vi "processMsg.vi"(8 "error in (no error)":errorcluster, 10 "Refs":refnum<vi>[](array[refnum]), 11 "Msg in":string) -> (0 "error out":errorcluster, 3 "Msg out":string)   [LabVIEW 2017]
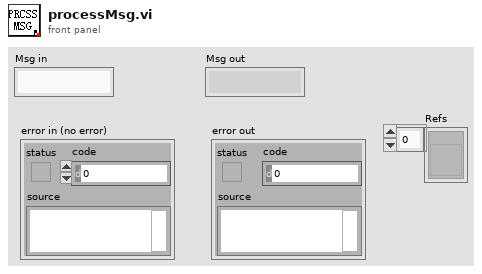
[diagram p1: front panel]
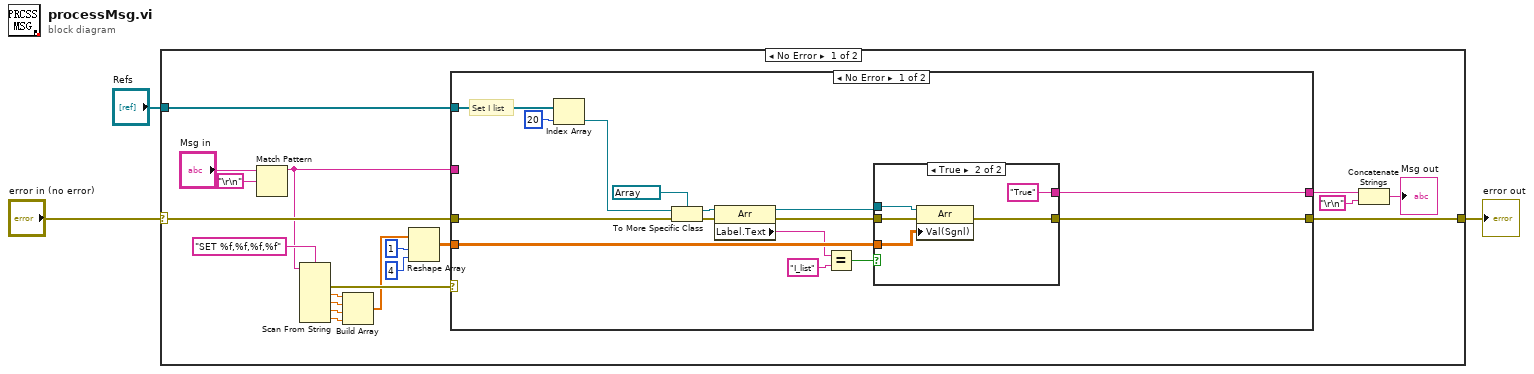
[diagram p0: block diagram]
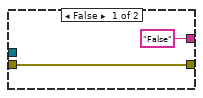
[diagram p2: hidden frame]
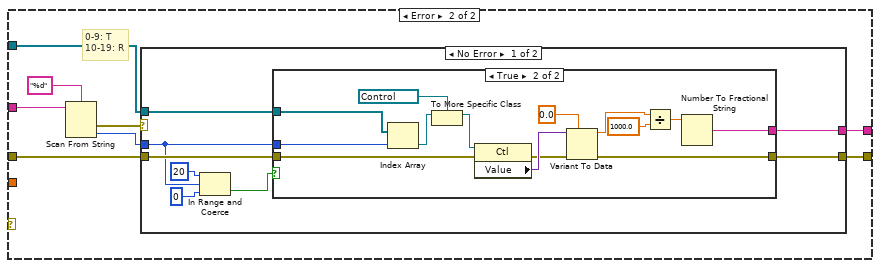
[diagram p3: hidden frame]
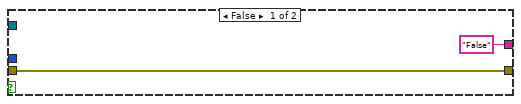
[diagram p4: hidden frame]
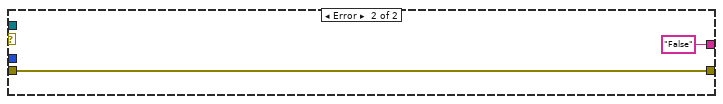
[diagram p5: hidden frame]
diagram:
  n1 = case shown="No Error" "error in (no error)" {
    selector: "error in (no error)" -> [w21 w79]
    tunnel: [w22 w79] -> w3
    tunnel: "Refs" -> [w15 _]
    frame No Error {
      n2 = Match Pattern(string="Msg in", regular expression="\r\n") -> (before substring=w17:string)  [unwired: 4 out]
      n3 = Scan From String(format string="SET %f,%f,%f,%f" ("regular expression"), input string=w17) -> (error out=w16:errorcluster, output 1=w14:dbl, output 2=w13:dbl, output 3=w12:dbl, output 4=w11:dbl)  [unwired: 6 in, 2 out]
      n4 = Build Array(w14, w13, w12, w11) -> (w10:dbl[])
      n5 = Reshape Array(w10, 1 ("dimension size"), 4 ("dimension size")) -> (w7:dbl[][])
      n6 = case shown="No Error" w16 {
        tunnel: [w23 w52] -> w22
        tunnel: w21 -> [w26 w47]
        tunnel: w17 -> [_ w49]
        tunnel: [w27 w51] -> w5
        tunnel: w15 -> [w37 w45]
        tunnel: w7 -> [w33 _]
        frame No Error {
          # "Set I list"
          n7 = Index Array(array=w37, index=20) -> (element=w34:refnum<vi>)
          n8 = To More Specific Class(target class=refnum<vi> refnum ("引用"), reference=w34, error in=w26) -> (specific class reference=w30:refnum<vi>, error out=w25:errorcluster)
          n9 = property class="Arr"(reference=w30, error in=w25) -> (reference out=w29:refnum<vi>, error out=w24:errorcluster, "Label.Text"=w31:string)
          n10 = Equal?(x=w31, y="I_list") -> (x = y?=w28:bool)
          n11 = case shown="True" w28 {
            tunnel: w33 -> [_ w44]
            tunnel: w29 -> [_ w43]
            tunnel: ["False" "True"] -> w27
            tunnel: w24 -> [w38 w41]
            tunnel: [w38 w40] -> w23
            frame False {
            }
            frame True {
              n12 = property class="Arr"(reference=w43, error in=w41, "Val(Sgnl)"=w44) -> (error out=w40:errorcluster)  [unwired: 1 out]
            }
          }
        }
        frame Error {
          # "0-9: T\n10-19: R"
          n13 = Scan From String(format string="%d" ("regular expression"), input string=w49) -> (error out=w48:errorcluster, output 1=w46:i32)  [unwired: 3 in, 2 out]
          n14 = case shown="No Error" w48 {
            tunnel: [w60 w78] -> w52
            tunnel: w47 -> [w59 w78]
            tunnel: [w58 "False" ("T (K) or R")] -> w51
            tunnel: w46 -> [w54 _]
            tunnel: w45 -> [w55 _]
            frame No Error {
              n15 = In Range and Coerce(upper limit=20, x=w54, lower limit=0) -> (In Range?=w53:bool)  [unwired: 1 out]
              n16 = case shown="True" w53 {
                tunnel: [w62 w65] -> w60
                tunnel: w59 -> [w62 w64]
                tunnel: ["False" ("T (K) or R") w63] -> w58
                tunnel: w55 -> [_ w70]
                tunnel: w54 -> [_ w69]
                frame False {
                }
                frame True {
                  n17 = Index Array(array=w70, index=w69) -> (element=w66:refnum<vi>)
                  n18 = To More Specific Class(target class=refnum<vi> refnum ("引用"), reference=w66) -> (specific class reference=w67:refnum<vi>)  [unwired: 1 in, 1 out]
                  n19 = property class="Ctl"(reference=w67, error in=w64) -> (error out=w72:errorcluster, "Value"=w73:variant)  [unwired: 1 out]
                  n20 = Variant To Data(error in=w72, type=0.0, Variant=w73) -> (data=w75:dbl, error out=w65:errorcluster)
                  n21 = Divide(x=w75, y=1000.0) -> (x/y=w71:dbl)
                  n22 = Number To Fractional String(number=w71) -> (F-format string=w63:string)  [unwired: 3 out]
                }
              }
            }
            frame Error {
            }
          }
        }
      }
      n23 = Concatenate Strings(w5, "\r\n") -> (→"Msg out":string)
    }
    frame Error {
    }
  }
  "error out" <- w3
